vi "get_task.vi"(8 "error in (no error)":errorcluster, 11 "DAQmxWriteSignals in":refnum<class "SignalWriterMM140725DAQmx.lvclass">) -> (0 "error out":errorcluster, 1 "index":i32, 2 "writer task":refnum<k21>, 3 "DAQmxWriteSignals out":refnum<class "SignalWriterMM140725DAQmx.lvclass">, 4 "found?":bool, 5 "counter task valid?":bool, 6 "counter task":refnum<k21>)   [LabVIEW 2010, in "SignalWriterMM140725DAQmx.lvclass"]
uses:
  SignalWriterMM140725DAQmx.lvclass
  <vilib>/regexp/Match Regular Expression.xnode
  Program Files (x86)/National Instruments/LabVIEW 2010/resource/objmgr/daqmx.rc
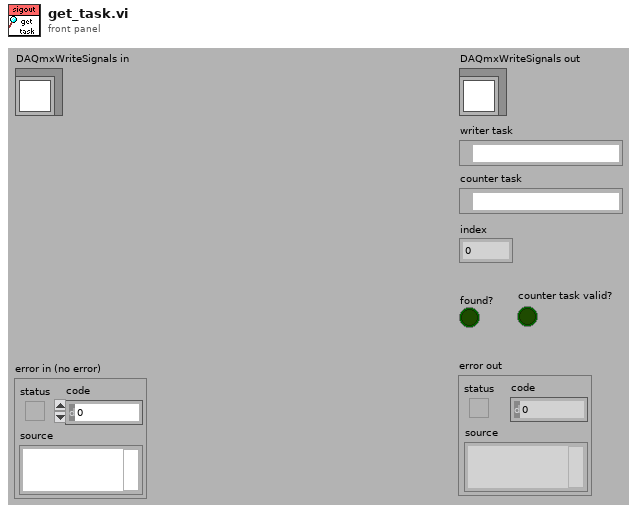
[diagram p1: front panel]
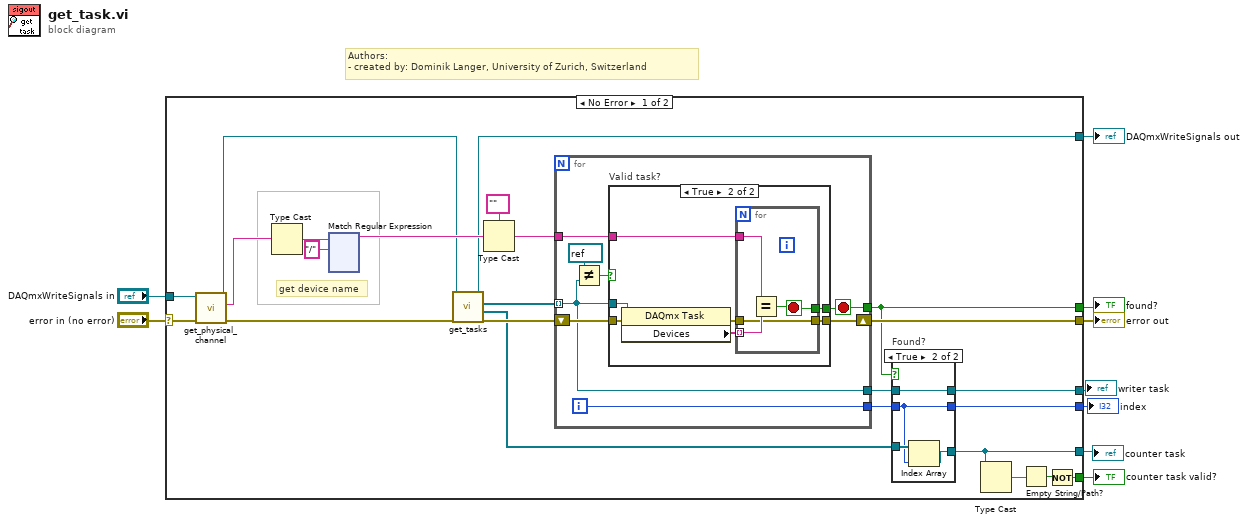
[diagram p0: block diagram]
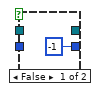
[diagram p2: hidden frame]
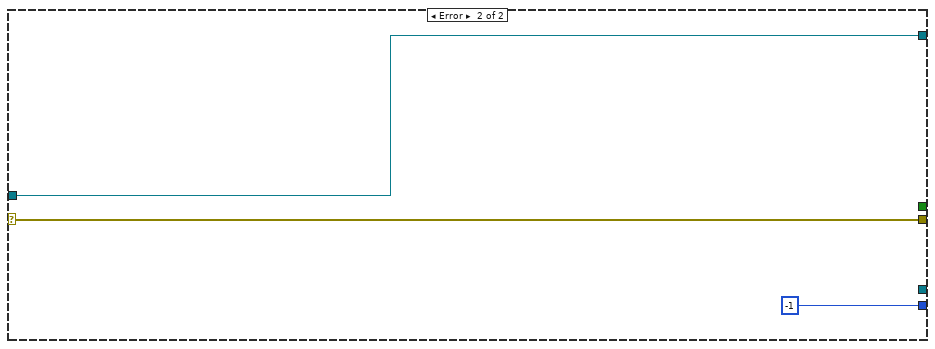
[diagram p4: hidden frame]
diagram:
  # "Authors: \n- created by: Dominik Langer, University of Zurich, Switzerland"
  n1 = case shown="No Error" "error in (no error)" {
    selector: "error in (no error)" -> [w19 w172]
    tunnel: [w28 w172] -> w8
    tunnel: [w20 w171] -> w6
    tunnel: "DAQmxWriteSignals in" -> [w16 w171]
    tunnel: [w27 _] -> w5
    tunnel: [w25 _] -> w4
    tunnel: [w23 -1] -> w3
    tunnel: [w13 _] -> w2
    tunnel: [w10 _] -> w1
    frame No Error {
      # "get device name"
      n2 = call-dynamic "get_physical_channel.vi"("error in (no error)"=w19, "DAQmxWriteSignals.lvclass in"=w16) -> ("error out"=w18:errorcluster, "physical channel"=w17:tag, "DAQmxWriteSignals.lvclass out"=w15:refnum<class "SignalWriterMM140725DAQmx.lvclass">)  [unwired: 7 out]
      n3 = Type Cast(x=w17) -> (*(type *) &x=w33:string)  [unwired: 1 out]
      n4 = xnode "Match Regular Expression"("input string"=w33, "regular expression"="/") -> ("before match"=w31:string)  [unwired: 2 in, 6 out]
      n5 = call-dynamic "get_tasks.vi"("error in (no error)"=w18, "DAQmxWriteSignals in"=w15) -> ("error out"=w22:errorcluster, "counter tasks"=w14:refnum<k21>[], "output tasks"=w21:refnum<k21>[], "DAQmxWriteSignals out"=w20:refnum<class "SignalWriterMM140725DAQmx.lvclass">)  [unwired: 6 out]
      n6 = Type Cast(type=tag "" ("DAQmx Device Name"), x=w31) -> (*(type *) &x=w30:tag)
      n7 = for {
        tunnel: w21 -> [w41] mode=indexing
        tunnel: w30 -> [w45]
        tunnel: [w44] -> w27
        tunnel: [w41] -> w26
        tunnel: [w42] -> w24
        shift-right: [w43] -> w28
        shift-left: w22 -> [w46]
        i -> [w42]
        stop <- w44 stop-if-true
        n8 = Not Equal?(x=refnum<k21> refnum ("analog output task"), y=w41) -> (x != y?=w39:bool)
        n9 = case "Valid task?" shown="True" w39 {
          tunnel: w46 -> [w47 w54]
          tunnel: w45 -> [_ w51]
          tunnel: [_ w50] -> w44
          tunnel: [w47 w49] -> w43
          tunnel: w41 -> [_ w48]
          frame False {
          }
          frame True {
            n10 = property class="DAQmx Task"(reference=w48, error in=w54) -> (error out=w53:errorcluster, "Devices"=w52:tag[])  [unwired: 1 out]
            n11 = for {
              tunnel: w53 -> [w55]
              tunnel: w52 -> [w57] mode=indexing
              tunnel: w51 -> [w58]
              tunnel: [w56] -> w50
              tunnel: [w55] -> w49
              stop <- w56 stop-if-true
              n12 = Equal?(x=w58, y=w57) -> (x = y?=w56:bool)
            }
          }
        }
      }
      n13 = case "Found?" shown="True" w27 {
        tunnel: [_ w38] -> w25
        tunnel: w26 -> [_ w38]
        tunnel: [-1 w36] -> w23
        tunnel: w24 -> [_ w36]
        tunnel: w14 -> [_ w37]
        tunnel: [_ w35] -> w13
        frame False {
        }
        frame True {
          n14 = Index Array(array=w37, index=w36) -> (element=w35:refnum<k21>)
        }
      }
      n15 = Type Cast(x=w13) -> (*(type *) &x=w12:string)  [unwired: 1 in]
      n16 = Empty String/Path?(string/path=w12) -> (empty?=w11:bool)
      n17 = Not(x=w11) -> (.not. x?=w10:bool)
    }
    frame Error {
    }
  }
  "error out" <- w8
  "DAQmxWriteSignals out" <- w6
  "writer task" <- w4
  "found?" <- w5
  "index" <- w3
  "counter task" <- w2
  "counter task valid?" <- w1
